vi "PR4000 cfg valve.vi"(8 "error in (no error)":errorcluster, 10 "Channel parsed command info":T1, 11 "MKS4000b in":refnum<class "ISSI_Iris.lvclass">) -> (0 "error out":errorcluster, 2 "new commands":string, 3 "MKS4000b out":refnum<class "ISSI_Iris.lvclass">)   [LabVIEW 2020]
uses:
  shared/CompressAndUpdate(Poly)/CompressAndUpdate(Enum).vi
  ISSI_Iris.lvclass
  C:/GEECS/Developers Version/source/Device Drivers/BaseDriver/BaseDriver.lvclass
  C:/GEECS/Developers Version/source/Device Drivers/ISSI_Iris/ISSI_Iris.lvclass
  Shared/Device Driver/channel parsed cmd cluster.ctl
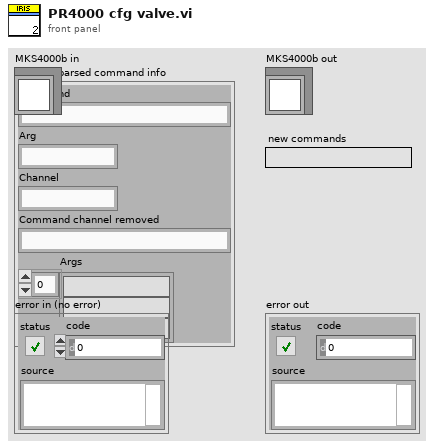
[diagram p1: front panel]
types:
  T1 = typedef "channel parsed cmd cluster.ctl" = cluster{"Command":string, "Arg":string, "Channel":string, "Command channel removed":string, "Args":string[]}
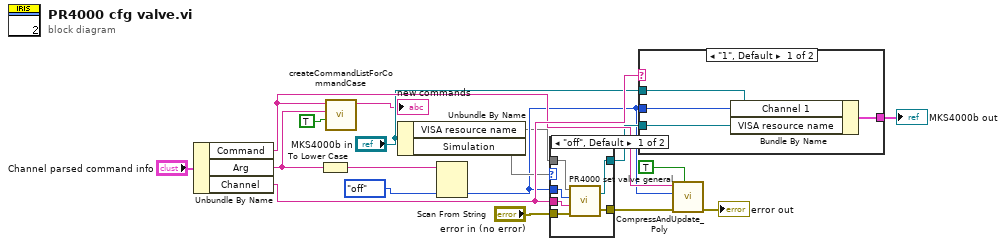
[diagram p0: block diagram]
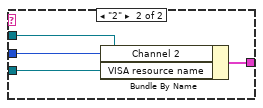
[diagram p3: hidden frame]
diagram:
  n1 = Unbundle By Name("Channel parsed command info") -> ("Command"=w16:string, "Arg"=w17:string, "Channel"=w18:string)
  n2 = To Lower Case(string=w17) -> (all lower case string=w10:string)
  n3 = call "createCommandListForCommandCase.vi"("immediate Check (only once)"=TRUE, "setvalue"=w17, "command"=w16) -> ("new commands"=→"new commands":string)  [unwired: 8 in]
  n4 = Unbundle By Name("MKS4000b in") -> ("VISA resource name"=w6, "Simulation"=w14)
  n5 = Scan From String(input string=w10, default 1=enum16{"off", "on"}."off" ("Settings.Save")) -> (output 1=w12:enum16{"off", "on"})  [unwired: 3 in, 3 out]
  n6 = case shown="\"off\", Default" w14 {
    tunnel: "error in (no error)" -> [w24 w25]
    tunnel: w6 -> [w23 w26]
    tunnel: [w22 w25] -> w11
    tunnel: w12 -> [w21 _]
    tunnel: [w20 w26] -> w13
    tunnel: w18 -> [w19 _]
    frame "off", Default {
      n7 = call "PR4000 set valve general.vi"("error"=w24, "channel no in"=w19, "Settings.Valve"=w21, "Comport PR4000"=w23) -> ("error out"=w22:errorcluster, "Comport PR4000 out"=w20:refnum<visa-resource-name>)
    }
    frame "on" {
    }
  }
  n8 = case shown="\"1\", Default" w18 {
    tunnel: [w30 w34] -> w1
    tunnel: "MKS4000b in" -> [w29 w33]
    tunnel: w12 -> [w28 w32]
    tunnel: w13 -> [w27 w31]
    frame "1", Default {
      n9 = Bundle By Name(cluster=w29, "Channel 1"=w28, "VISA resource name"=w27) -> (w30:cluster{})
    }
    frame "2" {
      n10 = Bundle By Name(cluster=w33, "Channel 2"=w32, "VISA resource name"=w31) -> (w34:cluster{})
    }
  }
  "MKS4000b out" <- w1
  n11 = call-poly "CompressAndUpdate_Poly.vi"("force CVT update (false)"=TRUE ("force CVT update"), "error in"=w11, "enum variant"=w12, "command or variable name"=w16) -> ("error out"=→"error out":errorcluster)  [unwired: 7 in]
